vi "XSens UTC (SubVI).vi"(0 "DATA In (Hex)":string) -> (1 "UTC Time":timestamp, 2 "UTC Time Status":T1={"Valid Time of Week"=TRUE, "Valid Week Number"=TRUE, "Valid UTC"=TRUE})   [LabVIEW 2019]
uses:
  <vilib>/Utility/miscctls.llb/LVDateTimeRec.ctl
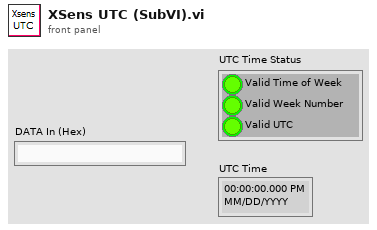
[diagram p1: front panel]
types:
  T1 = cluster{"Valid Time of Week":bool, "Valid Week Number":bool, "Valid UTC":bool}
  T2 = typedef "LVDateTimeRec.ctl" = cluster{"fractional second":dbl, "second":i32, "minute":i32, "hour":i32, "day of month":i32, "month":i32, "year":i32, "day of week":i32, "day of year":i32, "DST":i32}
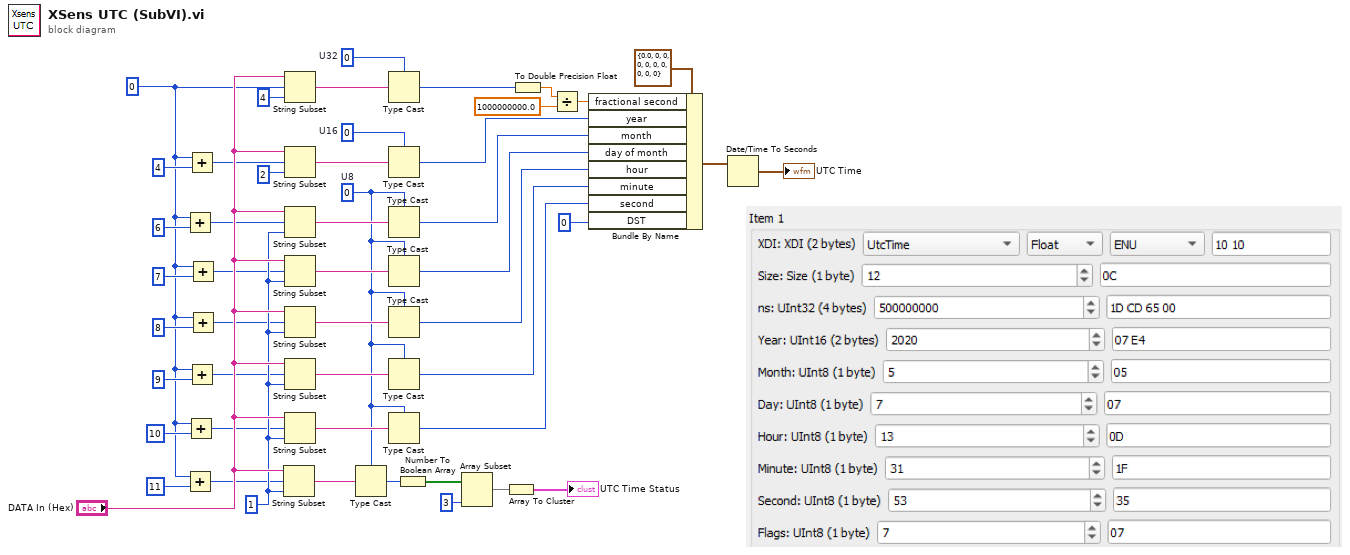
[diagram p0: block diagram]
diagram:
  w1 = 0
  w7 = 1 ("length (rest)")
  w40 = u32 0  # U32
  w42 = u16 0  # U16
  w17 = u8 0  # U8
  n1 = Add(x=w1, y=6 ("offset (0)")) -> (x+y=w13:i32)
  n2 = Add(x=w1, y=11 ("offset (0)")) -> (x+y=w2:i32)
  n3 = Add(x=w1, y=10 ("offset (0)")) -> (x+y=w3:i32)
  n4 = Add(x=w1, y=4 ("length (rest)")) -> (x+y=w15:i32)
  n5 = Add(x=w1, y=9 ("offset (0)")) -> (x+y=w4:i32)
  n6 = Add(x=w1, y=7 ("offset (0)")) -> (x+y=w6:i32)
  n7 = Add(x=w1, y=8 ("offset (0)")) -> (x+y=w5:i32)
  n8 = String Subset(string="DATA In (Hex)", offset (0)=w2, length (rest)=w7) -> (substring=w26:string)
  n9 = String Subset(string="DATA In (Hex)", offset (0)=w1, length (rest)=4 ("length (rest)")) -> (substring=w39:string)
  n10 = String Subset(string="DATA In (Hex)", offset (0)=w15, length (rest)=2 ("length (rest)")) -> (substring=w41:string)
  n11 = String Subset(string="DATA In (Hex)", offset (0)=w13, length (rest)=w7) -> (substring=w43:string)
  n12 = String Subset(string="DATA In (Hex)", offset (0)=w6, length (rest)=w7) -> (substring=w44:string)
  n13 = String Subset(string="DATA In (Hex)", offset (0)=w5, length (rest)=w7) -> (substring=w38:string)
  n14 = String Subset(string="DATA In (Hex)", offset (0)=w4, length (rest)=w7) -> (substring=w37:string)
  n15 = String Subset(string="DATA In (Hex)", offset (0)=w3, length (rest)=w7) -> (substring=w36:string)
  n16 = Type Cast(type=w17, x=w26) -> (*(type *) &x=w22:u8)
  n17 = Type Cast(type=w40, x=w39) -> (*(type *) &x=w19:u32)
  n18 = Type Cast(type=w42, x=w41) -> (*(type *) &x=w34:u16)
  n19 = Type Cast(type=w17, x=w43) -> (*(type *) &x=w33:u8)
  n20 = Type Cast(type=w17, x=w44) -> (*(type *) &x=w32:u8)
  n21 = Type Cast(type=w17, x=w38) -> (*(type *) &x=w31:u8)
  n22 = Type Cast(type=w17, x=w37) -> (*(type *) &x=w30:u8)
  n23 = Type Cast(type=w17, x=w36) -> (*(type *) &x=w29:u8)
  n24 = Number To Boolean Array(number=w22) -> (Boolean array=w25:bool[])
  n25 = Array Subset(array=w25, length=3) -> (w23:bool[])  [unwired: 1 in]
  n26 = Array To Cluster(array=w23) -> (cluster=→"UTC Time Status":cluster{"[0]":bool, "[1]":bool, "[2]":bool})
  n27 = To Double Precision Float(number=w19) -> (double precision float=w18:dbl)
  n28 = Divide(x=w18, y=1000000000.0) -> (x/y=w20:dbl)
  n29 = Bundle By Name(cluster=T2 {"fractional second"=0.0, "second"=0, "minute"=0, "hour"=0, "day of month"=0, "month"=0, "year"=0, "day of week"=0, "day of year"=0, "DST"=0} ("date time rec"), "fractional second"=w20, "year"=w34, "month"=w33, "day of month"=w32, "hour"=w31, "minute"=w30, "second"=w29, "DST"=0) -> (w28:T2)
  n30 = Date/Time To Seconds(2:w28) -> (0:→"UTC Time":timestamp)  [unwired: 1 in]
